vi "Enqueue Multiple States.vi"(0 "State(s) at Front":string, 5 "queue in":refnum<queue>, 7 "State(s) at Back":string) -> (6 "queue out":refnum<queue>)   [LabVIEW 2020, in "VI Properties Editor.lvlib"]
doc: "Adds states to the front and/or back of the queue. Use \"Enqueue Element.vi\" and \"Enqueue Element at Opposite End.vi\" instead of this if there is data to be bundled with the state.\n\nCurrently, if this is used to enqueue multiple states at the opposite end from the Producer Loop, unexpected behavior can result."
uses:
  VI Properties Editor.lvlib
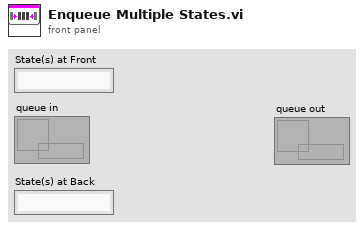
[diagram p1: front panel]
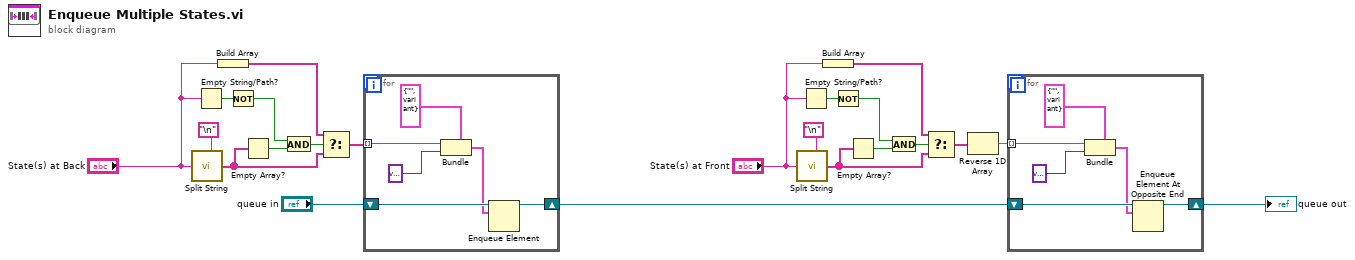
[diagram p0: block diagram]
diagram:
  n1 = call <vilib>:"Split String.vi"("Split Pattern"="\n", "Input String"="State(s) at Back") -> ("Split String"=w18:string[])  [unwired: 5 in]
  n2 = Empty String/Path?(string/path="State(s) at Back") -> (empty?=w14:bool)
  n3 = Build Array("State(s) at Back") -> (w17:string[])
  n4 = Not(x=w14) -> (.not. x?=w13:bool)
  n5 = Empty Array?(array=w18) -> (empty?=w12:bool)
  n6 = And(x=w13, y=w12) -> (x .and. y?=w11:bool)
  n7 = Select(t=w17, s=w11, f=w18) -> (s? t:f=w16:string[])
  n8 = for {
    tunnel: w16 -> [w27] mode=indexing
    shift-right: [w24] -> w19
    shift-left: "queue in" -> [w25]
    n9 = Bundle(cluster=cluster{string, variant} {"", variant} ("element"), w27, variant) -> (w23:cluster{string, variant})
    n10 = Enqueue Element(queue=w25, element=w23) -> (queue out=w24:refnum<queue>)  [unwired: 2 in, 2 out]
  }
  n11 = call <vilib>:"Split String.vi"("Split Pattern"="\n", "Input String"="State(s) at Front") -> ("Split String"=w5:string[])  [unwired: 5 in]
  n12 = Empty String/Path?(string/path="State(s) at Front") -> (empty?=w7:bool)
  n13 = Build Array("State(s) at Front") -> (w6:string[])
  n14 = Not(x=w7) -> (.not. x?=w8:bool)
  n15 = Empty Array?(array=w5) -> (empty?=w9:bool)
  n16 = And(x=w8, y=w9) -> (x .and. y?=w10:bool)
  n17 = Select(t=w6, s=w10, f=w5) -> (s? t:f=w2:string[])
  n18 = Reverse 1D Array(array=w2) -> (reversed array=w20:string[])
  n19 = for {
    tunnel: w20 -> [w33] mode=indexing
    shift-right: [w30] -> w1
    shift-left: w19 -> [w31]
    n20 = Bundle(cluster=cluster{string, variant} {"", variant} ("element"), w33, variant) -> (w29:cluster{string, variant})
    n21 = Enqueue Element At Opposite End(queue=w31, element=w29) -> (queue out=w30:refnum<queue>)  [unwired: 2 in, 2 out]
  }
  "queue out" <- w1
